vi "3d model graph.vi"() -> ()   [LabVIEW 2012]
uses:
  <vilib>/Utility/miscctls.llb/LV3DPointTypeDef.ctl
  <vilib>/picture/3D Picture Control/NI_3D Picture Control.lvlib
panel:
  in  "Translation":T1
  in  "Z":sgl step=0.1
  in  "default Y":sgl step=0.1
  in  "default X":sgl step=0.1
  in  "stop":bool
  in  "STL File Path":path
  out "3D Picture Control":refnum<vi>(3d-picture)
  # "DEFAULT"
  # "Axis"
  # "Translation"
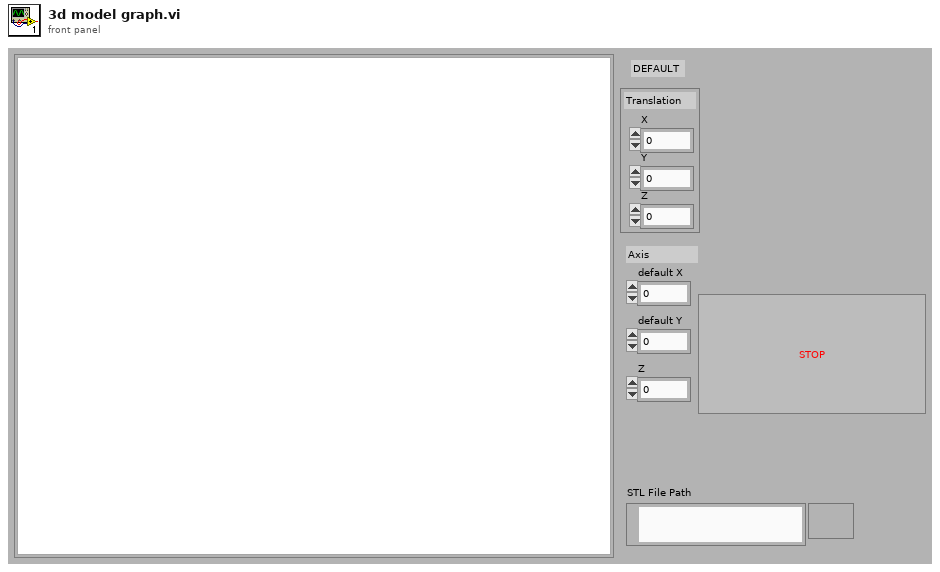
[diagram p1: front panel]
types:
  T1 = typedef "LV3DPointTypeDef.ctl" = cluster{"X":sgl, "Y":sgl, "Z":sgl}
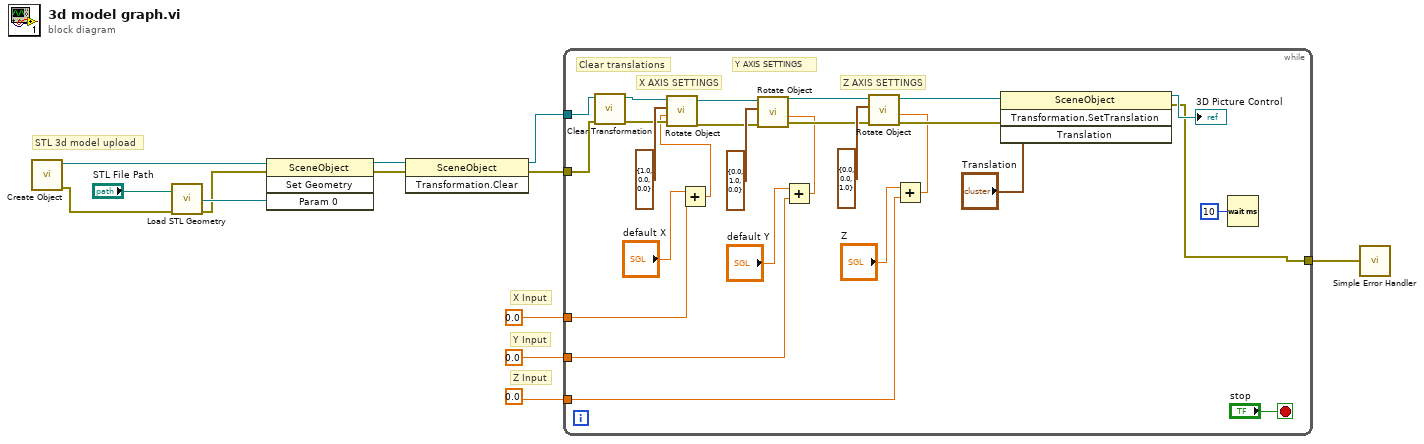
[diagram p0: block diagram]
diagram:
  # "STL 3d model upload"
  # "Z Input"
  # "Y Input"
  # "X Input"
  n1 = call <vilib>:"Create Object.vi"() -> ("error out"=w12:errorcluster, "Scene:New Object"=w10:refnum<vi>)  [unwired: 2 in, 8 out]
  n2 = call <vilib>:"Load STL Geometry.vi"("error in (no error)"=w12, "Model File"="STL File Path") -> ("error out"=w9:errorcluster, "New Mesh Refnum"=w11:refnum<vi>)  [unwired: 8 out]
  n3 = invoke class="SceneObject" method="Set Geometry"(reference=w10, error in=w9, "Param 0"=w11) -> (reference out=w7:refnum<vi>, error out=w6:errorcluster)  [unwired: 1 in, 2 out]
  n4 = invoke class="SceneObject" method="Transformation.Clear"(reference=w7, error in=w6) -> (reference out=w5:refnum<vi>, error out=w4:errorcluster)  [unwired: 1 in, 1 out]
  n5 = while {
    tunnel: [w24] -> w8
    tunnel: w5 -> [w36]
    tunnel: w4 -> [w35]
    tunnel: sgl 0.0 ("y") -> [w20]
    tunnel: sgl 0.0 ("y") -> [w18]
    tunnel: sgl 0.0 ("y") -> [w15]
    stop <- "stop" stop-if-true
    # "Z AXIS SETTINGS"
    # "Y AXIS SETTINGS"
    # "Clear translations"
    # "X AXIS SETTINGS"
    n6 = call <vilib>:"Clear Transformation.vi"("error in (no error)"=w35, "Object Refnum In"=w36) -> ("error out"=w25:errorcluster, "Object Refnum Out"=w37:refnum<vi>)  [unwired: 8 out]
    n7 = Add(x="default X", y=w20) -> (x+y=w22:sgl)
    n8 = call <vilib>:"Rotate Object.vi"("error in (no error)"=w25, "Angle"=w22, "Axis"=cluster{"X":sgl, "Y":sgl, "Z":sgl} {"X"=1.0, "Y"=0.0, "Z"=0.0}, "Scene.Object In"=w37) -> ("error out"=w26:errorcluster, "Scene.Object Out"=w27:refnum<vi>)  [unwired: 6 out]
    n9 = Add(x="default Y", y=w18) -> (x+y=w17:sgl)
    n10 = call <vilib>:"Rotate Object.vi"("error in (no error)"=w26, "Angle"=w17, "Axis"=cluster{"X":sgl, "Y":sgl, "Z":sgl} {"X"=0.0, "Y"=1.0, "Z"=0.0}, "Scene.Object In"=w27) -> ("error out"=w28:errorcluster, "Scene.Object Out"=w29:refnum<vi>)  [unwired: 6 out]
    n11 = Add(x="Z", y=w15) -> (x+y=w14:sgl)
    n12 = call <vilib>:"Rotate Object.vi"("error in (no error)"=w28, "Angle"=w14, "Axis"=cluster{"X":sgl, "Y":sgl, "Z":sgl} {"X"=0.0, "Y"=0.0, "Z"=1.0}, "Scene.Object In"=w29) -> ("error out"=w30:errorcluster, "Scene.Object Out"=w31:refnum<vi>)  [unwired: 6 out]
    n13 = invoke class="SceneObject" method="Transformation.SetTranslation"(reference=w31, error in=w30, "Translation"="Translation") -> (reference out=→"3D Picture Control":refnum<vi>, error out=w24:errorcluster)  [unwired: 1 in, 2 out]
    n14 = Wait (ms)(milliseconds to wait=u32 10) -> ()  [unwired: 1 out]
  }
  n15 = call <vilib>:"Simple Error Handler.vi"("error in (no error)"=w8) -> ()  [unwired: 1 in, 8 out]
